vi "DAQDigitalTask.vi"() -> (0 "error out":errorcluster, 1 "Expected Signal Read":bool, 2 "data":digitalwaveform(waveform)={"t0"=timestamp(0 s since 1904-01-01), "dt"=0.0, "Y"={"transitions"=[], "data"=[]}, "error"={"status"=FALSE, "code"=37421928, "source"=""}})   [LabVIEW 2011]
uses:
  <vilib>/DAQmx/read.llb/DAQmx Read (Digital Wfm 1Chan NSamp).vi
  <vilib>/DAQmx/miscellaneous.llb/DAQmx Fill In Error Info.vi
panel:
  in  "Expected values":digitaldata={"transitions"=[], "data"=[[0], [1], [0], [1], [0], [1], [0], [1], [0], [1], [0], [1], [0], [1], [0], [1], [0], [1], [0], [1], [0], [1], [0], [1], [0], [1], [0], [1], [0], [1], [0], [1], [0], [1], [0], [1], [0], [1], [0], [1], [0], [1], [0], [1], [0], [1], [0], [1], [0], [1], [0], [1], [0], [1], [0], [1], [0], [1], [0], [1], [0], [1], [0], [1], [0], [1], [0], [1], [0], [1], [0], [1], [0], [1], [0], [1], [0], [1], [0], [1], [0], [1], [0], [1], [0], [1], [0], [1], [0], [1], [0], [1], [0], [1], [0], [1], [0], [1], [0], [1]]}
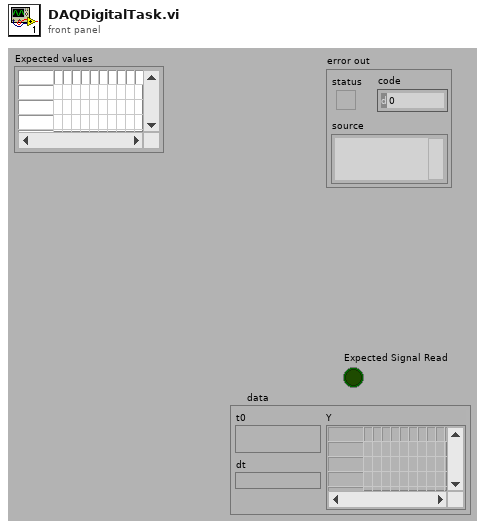
[diagram p1: front panel]
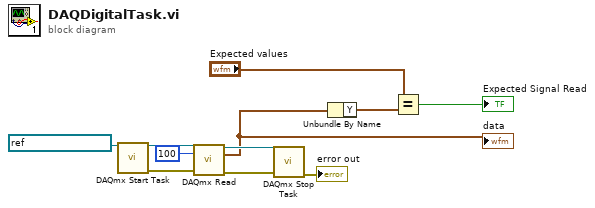
[diagram p0: block diagram]
diagram:
  n1 = call <vilib>:"DAQmx Start Task.vi"("task/channels in"=refnum<k21> "MyDigitalInTask") -> ("task out"=w10:refnum<k21>, "error out"=w9:errorcluster)  [unwired: 13 in]
  n2 = call-poly <vilib>:"DAQmx Read.vi"("task/channels in"=w10, "number of samples per channel"=100, "error in"=w9) -> ("task out"=w7:refnum<k21>, "data"=w3:digitalwaveform, "error out"=w8:errorcluster)  [unwired: 10 in]
  "data" <- w3
  n3 = call <vilib>:"DAQmx Stop Task.vi"("task/channels in"=w7, "error in"=w8) -> ("error out"=→"error out":errorcluster)  [unwired: 12 in, 1 out]
  n4 = Unbundle By Name(w3) -> ("Y"=w2:digitaldata)
  n5 = Equal?(x="Expected values", y=w2) -> (x = y?=→"Expected Signal Read":bool)
